vi "1-4.vi"() -> ()   [LabVIEW 2022 SP3]
panel:
  out "随机数":dbl format="%.2f"
  out "相乘结果":dbl format="%.2f"
  out "最终结果":dbl format="%.2f"
  # "程序功能：\n（1）产生一个随机数与10.0相乘，\n（2）然后通过一个VI子程序将积与100相加后开方。"
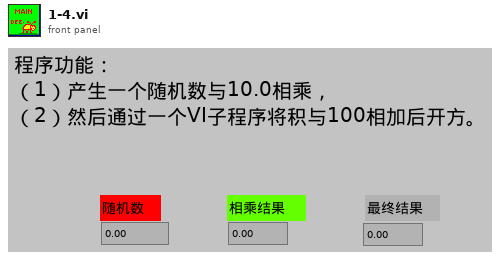
[diagram p1: front panel]
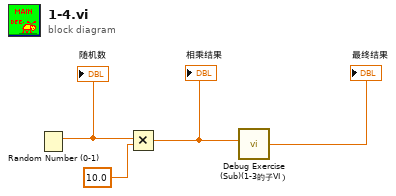
[diagram p0: block diagram]
diagram:
  n1 = Random Number (0-1)() -> (number: 0 to 1=w2:dbl)
  "随机数" <- w2
  n2 = Multiply(x=w2, y=10.0) -> (x*y=w4:dbl)
  "相乘结果" <- w4
  n3 = call "Debug Exercise (Sub)(1-3的子VI）.vi"("Number"=w4) -> ("Final Result"=→"最终结果":dbl)
